vi "Valves about to Open.vi"(8 "error in (no error)":errorcluster, 9 "timeout in ms (-1)":i32=-1, 10 "Requested Bit Field":u16, 11 "Storage Line in":refnum<class "Storage Line.lvclass">) -> (0 "error out":errorcluster, 1 "Boolean array of valves about to Open":bool[](array[boolean]), 2 "Bitfield of valves about to Open":u16, 3 "Storage Line out":refnum<class "Storage Line.lvclass">)   [LabVIEW 2015, in "cRIO-Carbondioxide.lvlib" / "CO2-Actor.lvlib" / "Storage Line.lvclass"]
uses:
  Storage Line.lvclass
  Storage Line.lvclass/Storage Line.ctl
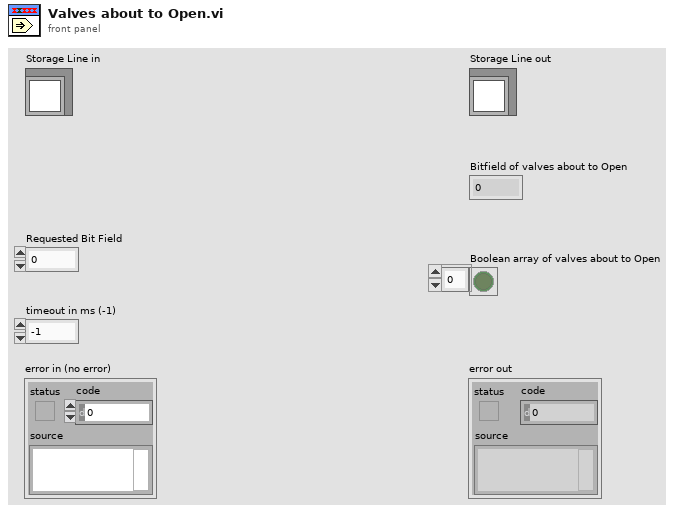
[diagram p1: front panel]
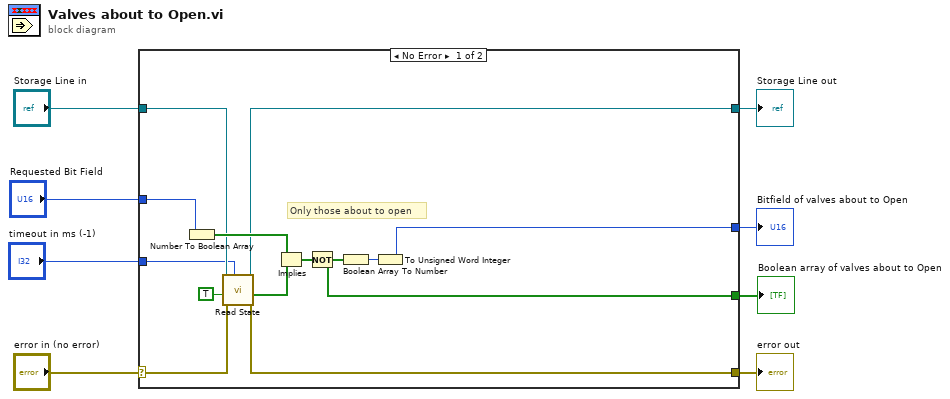
[diagram p0: block diagram]
diagram:
  n1 = case shown="No Error" "error in (no error)" {
    selector: "error in (no error)" -> [w15 w23]
    tunnel: [w12 w23] -> w7
    tunnel: [w13 w22] -> w5
    tunnel: "Storage Line in" -> [w14 w22]
    tunnel: "Requested Bit Field" -> [w16 _]
    tunnel: "timeout in ms (-1)" -> [w11 _]
    tunnel: [w10 _] -> w2
    tunnel: [w9 _] -> w1
    frame No Error {
      # "Only those about to open"
      n2 = Number To Boolean Array(number=w16) -> (Boolean array=w18:bool[])
      n3 = call "Read State.vi"("timeout in ms (-1)"=w11, "error in (no error)"=w15, "Return Boolean Array? (F)"=TRUE, "Storage Line in"=w14) -> ("error out"=w12:errorcluster, "Boolean array"=w20:bool[], "Storage Line out"=w13:refnum<class "Storage Line.lvclass">)  [unwired: 3 in, 2 out]
      n4 = Implies(1:w20, 2:w18) -> (0:w19:bool[])
      n5 = Not(x=w19) -> (.not. x?=w10:bool[])
      n6 = Boolean Array To Number(Boolean array=w10) -> (number=w17:u32)
      n7 = To Unsigned Word Integer(number=w17) -> (unsigned 16bit integer=w9:u16)
    }
    frame Error {
    }
  }
  "error out" <- w7
  "Storage Line out" <- w5
  "Boolean array of valves about to Open" <- w2
  "Bitfield of valves about to Open" <- w1
